vi "check_Coh_Faktor_past_Values.vi"(10 "Coh Faktor Thresold in":dbl, 11 "Array":dbl[](array[numeric])) -> (3 "Boolean":bool)   [LabVIEW 2018]
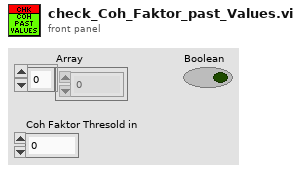
[diagram p1: front panel]
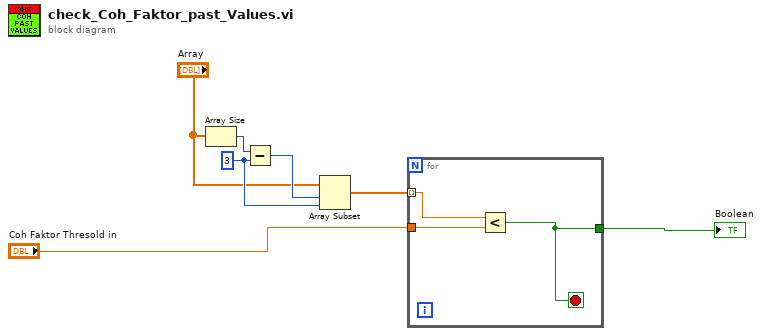
[diagram p0: block diagram]
diagram:
  w4 = 3 ("y")
  n1 = Array Size(array="Array") -> (size(s)=w2:i32)
  n2 = Subtract(x=w2, y=w4) -> (x-y=w3:i32)
  n3 = Array Subset(array="Array", index=w3, length=w4) -> (w5:dbl[])
  n4 = for {
    tunnel: w5 -> [w10] mode=indexing
    tunnel: "Coh Faktor Thresold in" -> [w9]
    tunnel: [w8] -> w7
    stop <- w8 stop-if-true
    n5 = Less?(x=w10, y=w9) -> (x < y?=w8:bool)
  }
  "Boolean" <- w7
